vi "test.file.xml.vi"() -> ()   [LabVIEW 2017]
panel:
  out "TAG":string
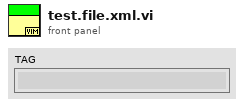
[diagram p1: front panel]
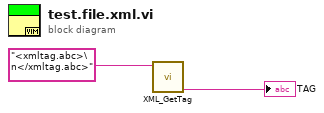
[diagram p0: block diagram]
diagram:
  n1 = call "XML_GetTag.vi"("XML"="<xmltag.abc>\n</xmltag.abc>") -> ("TAG"=→"TAG":string)  [unwired: 9 in, 1 out]
